vi "GetDigitalConstructor.vi"(6 "error in":errorcluster, 9 "Control in":refnum<class "Digital.lvclass">) -> (0 "error out":errorcluster, 3 "Control out":refnum<class "Digital.lvclass">, 4 "constructor":string, 5 "module":T1)   [LabVIEW 2014, in "PythonConverter_GUI.lvclass"]
uses:
  PythonConverter_GUI.lvclass
  VI Interpreter/Classes/Digital/Digital.lvclass
  TypeDefs/PythonModuleTD.ctl
  VI Interpreter/Classes/Control/Control.lvclass
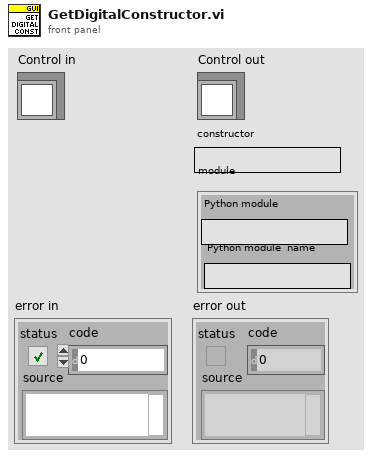
[diagram p1: front panel]
types:
  T1 = typedef "PythonConverter_GUI.lvclass/PythonModuleTD.ctl" = cluster{"Python module":string, "Python module  name":string}
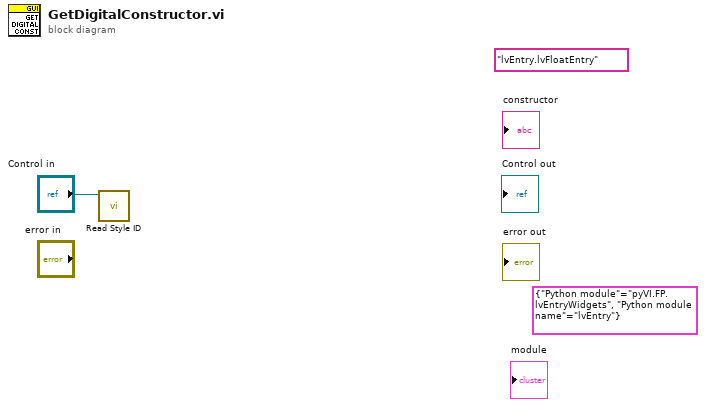
[diagram p0: block diagram]
diagram:
  (unwired) T1 {"Python module"="pyVI.FP.lvEntryWidgets", "Python module  name"="lvEntry"} ("module")
  (unwired) "lvEntry.lvFloatEntry"
  n1 = call "Read Style ID.vi"("Control in"="Control in") -> ()  [unwired: 7 in, 2 out]
